vi "Initialize Logging.vi"(8 "error in (no error)":errorcluster, 11 "Logging Configuration":T1) -> (0 "error out":errorcluster, 3 "Logging Configuration Out":T1)   [LabVIEW 2013, in "Logging.lvlib"]
uses:
  Logging.lvlib
  Logging Configuration.ctl
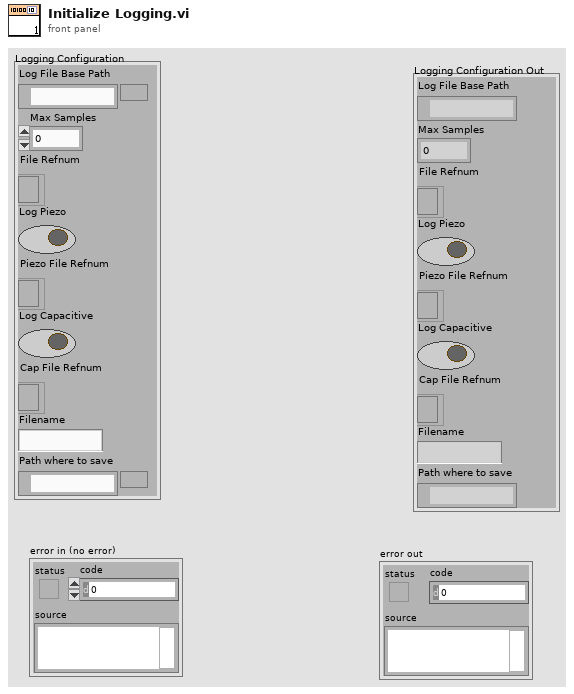
[diagram p1: front panel]
types:
  T1 = typedef "Logging.lvlib/Logging Configuration.ctl" = cluster{"Log File Base Path":path, "Max Samples":u32, "File Refnum":refnum<file>, "Log Piezo":bool, "Piezo File Refnum":refnum<file>, "Log Capacitive":bool, "Cap File Refnum":refnum<file>, "Filename":string, "Path where to save":path}
  T2 = enum16{"open", "replace", "create", "open or create", "replace or create", "replace or create with confirmation"}
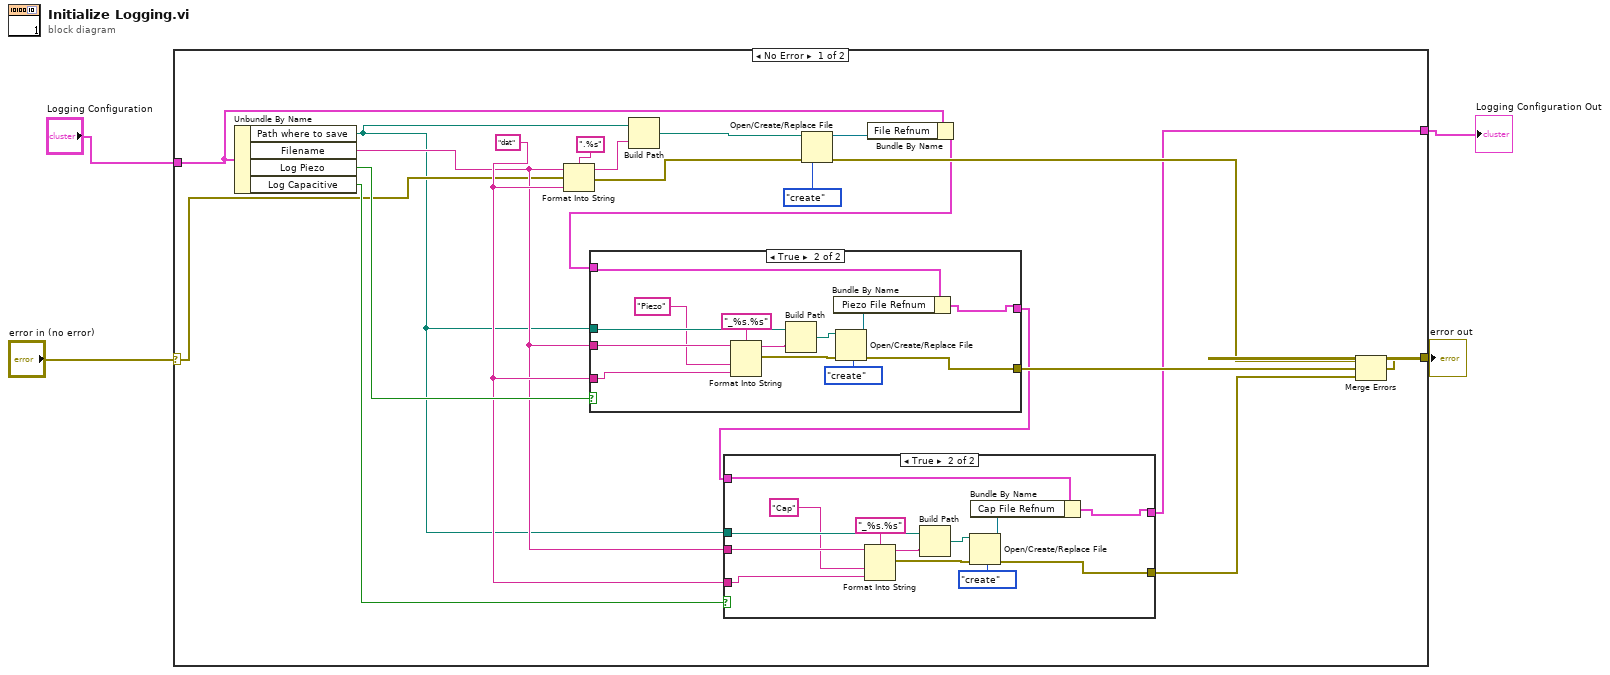
[diagram p0: block diagram]
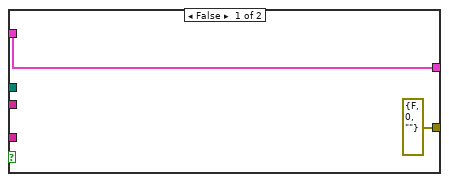
[diagram p2: hidden frame]
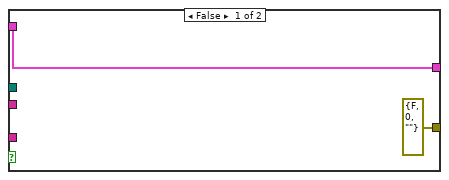
[diagram p3: hidden frame]
diagram:
  n1 = case shown="No Error" "error in (no error)" {
    selector: "error in (no error)" -> [w6 w55]
    tunnel: "Logging Configuration" -> [w18 w56]
    tunnel: [w10 w56] -> w3
    tunnel: [w17 w55] -> w2
    frame No Error {
      w8 = "dat" ("format string")
      n2 = Unbundle By Name(w18) -> ("Path where to save"=w5:path, "Filename"=w7:string, "Log Piezo"=w16:bool, "Log Capacitive"=w9:bool)
      n3 = Format Into String(format string=".%s", initial string=w7, error in=w6, w8) -> (resulting string=w20:string, error out=w13:errorcluster)
      n4 = Build Path(base path=w5, name or relative path=w20) -> (appended path=w22:path)
      n5 = Open/Create/Replace File(file path (use dialog)=w22, error in=w13, operation (0:open)=T2."create") -> (refnum out=w24:refnum<file>, error out=w21:errorcluster)  [unwired: 3 in, 1 out]
      n6 = Bundle By Name(cluster=w18, "File Refnum"=w24) -> (w15:T1)
      n7 = case shown="True" w16 {
        tunnel: w5 -> [_ w49]
        tunnel: w7 -> [_ w48]
        tunnel: w8 -> [_ w47]
        tunnel: w15 -> [w41 w45]
        tunnel: [w41 w44] -> w12
        tunnel: [errorcluster {"status"=FALSE, "code"=0, "source"=""} ("error out") w43] -> w14
        frame False {
        }
        frame True {
          n8 = Format Into String(format string="_%s.%s", initial string=w48, "Piezo" ("input 2"), w47) -> (resulting string=w51:string, error out=w42:errorcluster)  [unwired: 1 in]
          n9 = Build Path(base path=w49, name or relative path=w51) -> (appended path=w52:path)
          n10 = Open/Create/Replace File(file path (use dialog)=w52, error in=w42, operation (0:open)=T2."create") -> (refnum out=w54:refnum<file>, error out=w43:errorcluster)  [unwired: 3 in, 1 out]
          n11 = Bundle By Name(cluster=w45, "Piezo File Refnum"=w54) -> (w44:T1)
        }
      }
      n12 = case shown="True" w9 {
        tunnel: w5 -> [_ w34]
        tunnel: w7 -> [_ w33]
        tunnel: w8 -> [_ w32]
        tunnel: w12 -> [w26 w30]
        tunnel: [w26 w29] -> w10
        tunnel: [errorcluster {"status"=FALSE, "code"=0, "source"=""} ("error out") w28] -> w11
        frame False {
        }
        frame True {
          n13 = Format Into String(format string="_%s.%s", initial string=w33, "Cap" ("input 2"), w32) -> (resulting string=w36:string, error out=w27:errorcluster)  [unwired: 1 in]
          n14 = Build Path(base path=w34, name or relative path=w36) -> (appended path=w37:path)
          n15 = Open/Create/Replace File(file path (use dialog)=w37, error in=w27, operation (0:open)=T2."create") -> (refnum out=w39:refnum<file>, error out=w28:errorcluster)  [unwired: 3 in, 1 out]
          n16 = Bundle By Name(cluster=w30, "Cap File Refnum"=w39) -> (w29:T1)
        }
      }
      n17 = Merge Errors(w21, w14, w11) -> (w17:errorcluster)
    }
    frame Error {
    }
  }
  "Logging Configuration Out" <- w3
  "error out" <- w2
